vi "Scale.vi"(8 "error in":errorcluster, 10 "Input":variant, 11 "Scaling Strategy in":refnum<class "Scaling Strategy.lvclass">) -> (0 "error out":errorcluster, 2 "Output":variant, 3 "Scaling Strategy out":refnum<class "Scaling Strategy.lvclass">)   [LabVIEW 2024, in "HAL.lvlib" / "Scaling Strategy.lvclass"]
uses:
  Scaling Strategy.lvclass
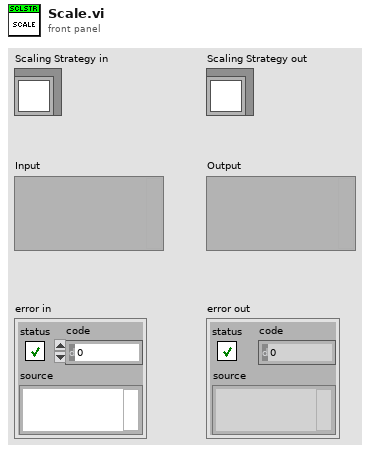
[diagram p1: front panel]
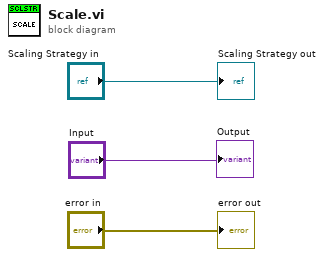
[diagram p0: block diagram]
diagram:
  "error out" <- "error in"
  "Scaling Strategy out" <- "Scaling Strategy in"
  "Output" <- "Input"
